vi "GetEdge DetectionResultValue.vi"(8 "error in (no error)":errorcluster, 9 "data":T2 {"Edge Information"."Distance (Real-World)" format="%.2f"; "Edge Information"."Location (Real-World)"."Y" format="%.2g"; "Edge Information"."Location (Real-World)"."X" format="%.2f"; "Edge Information"."Noise" format="%.2f"; "Edge Information"."Location (Pixel)"."Y" format="%.2g"; "Edge Information"."Location (Pixel)"."X" format="%.2f"; "Edge Information"."Strength" format="%.2f"; "Edge Information"."Distance (Pixel)" format="%.2f"}, 11 "Analysis_Edge Detection_Parameter":T3={"Edge Options"={"Edge Polarity"=0, "Kernel Size"=3, "Width"=5, "Minimum Edge Strength"=10.0, "Interpolation Type"=1, "Data Processing Method"=0}, "Process"=2, "Number of Matches Requested"=1, "ROI Descriptor"={"Global Rectangle"=[], "Contours"=[]}} {"Process" items=["Get First Edge", "Get First + Last Edge", "Get All Edges", "Get Best Edge"]; "Edge Options"."Data Processing Method" items=["Average", "Median"]; "Edge Options"."Interpolation Type" items=["Zero Order"=0, "Bilinear"=1, "Bilinear Fixed"=4]; "Edge Options"."Minimum Edge Strength" min=0.0 max=255.0 format="%.2g"; "Edge Options"."Width" min=1 step=2; "Edge Options"."Kernel Size" min=3 step=2; "Edge Options"."Edge Polarity" items=["All Edges", "Rising Edges", "Falling Edges"]}) -> (0 "error out":errorcluster, 3 "ResultValues":string[](array[string]))   [LabVIEW 2019]
uses:
  Controls/Edge Detection/Analysis_Edge Detection_Parameter.ctl
  <vilib>/vision/Measure.llb/Edge New.ctl
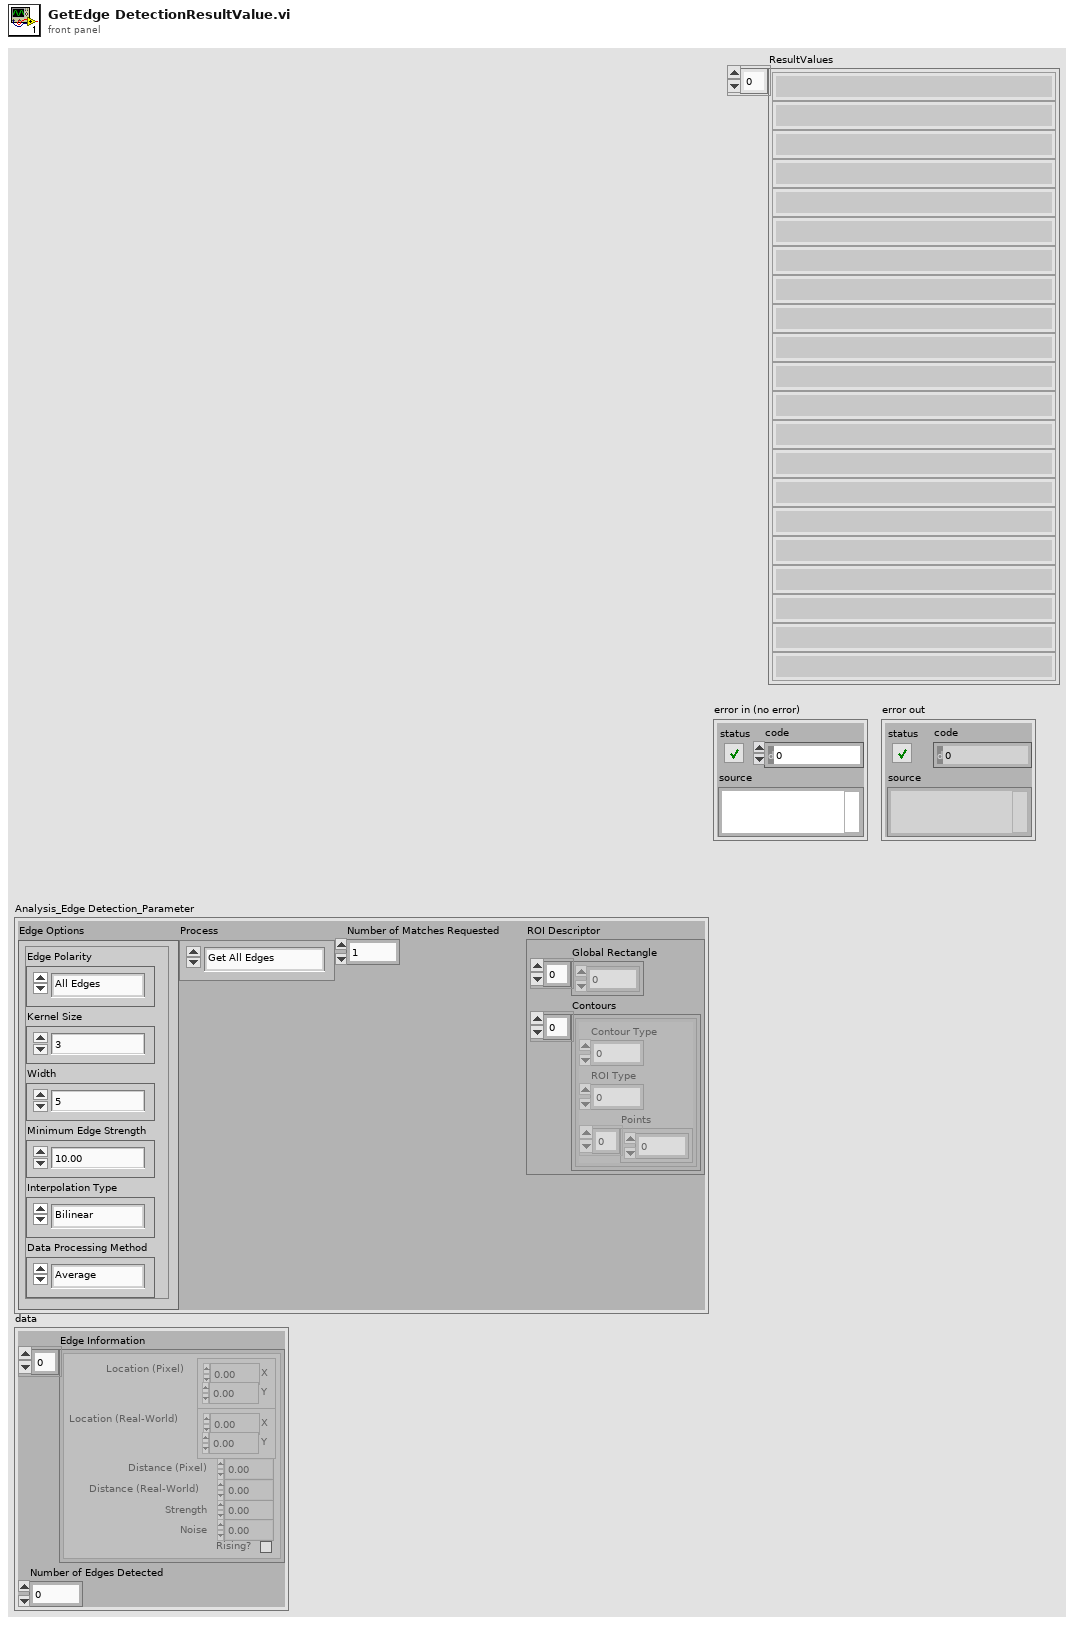
[diagram p1: front panel]
types:
  T1 = typedef "Edge New.ctl" = cluster{"Location (Pixel)":cluster{"X":sgl, "Y":sgl}, "Location (Real-World)":cluster{"X":sgl, "Y":sgl}, "Distance (Pixel)":dbl, "Distance (Real-World)":dbl, "Strength":dbl, "Noise":dbl, "Rising?":bool}
  T2 = cluster{"Edge Information":T1[], "Number of Edges Detected":i32}
  T3 = typedef "Analysis_Edge Detection_Parameter.ctl" = cluster{"Edge Options":cluster{"Edge Polarity":u16, "Kernel Size":u32, "Width":u32, "Minimum Edge Strength":dbl, "Interpolation Type":u16, "Data Processing Method":u16}, "Process":u16, "Number of Matches Requested":i32, "ROI Descriptor":cluster{"Global Rectangle":i32[], "Contours":cluster{"Contour Type":u32, "ROI Type":u32, "Points":i32[]}[]}}
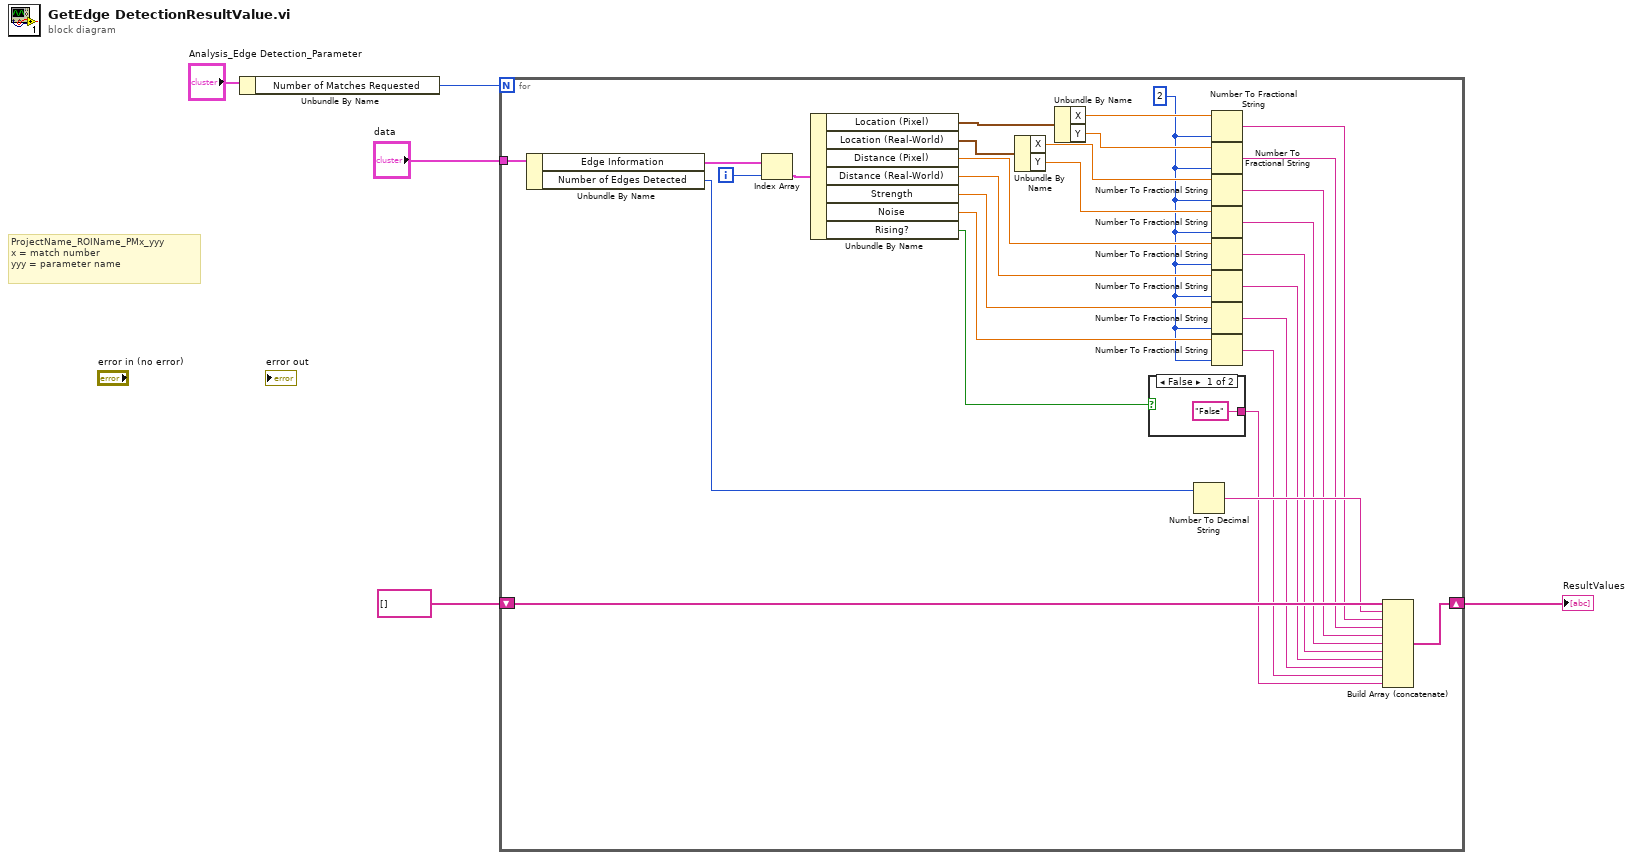
[diagram p0: block diagram]
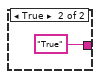
[diagram p2: hidden frame]
diagram:
  # "ProjectName_ROIName_PMx_yyy\nx = match number\nyyy = parameter name"
  n1 = Unbundle By Name("Analysis_Edge Detection_Parameter") -> ("Number of Matches Requested"=w2:i32)
  n2 = for {
    N: w2 -> [_]
    shift-right: [w8] -> w4
    shift-left: string[] [] -> [w18]
    tunnel: "data" -> [w34]
    i -> [w32]
    w6 = 2
    n3 = Unbundle By Name(w34) -> ("Edge Information"=w33:T1[], "Number of Edges Detected"=w30:i32)
    n4 = Index Array(array=w33, index=w32) -> (element=w31:T1)
    n5 = Unbundle By Name(w31) -> ("Location (Pixel)"=w29:cluster{"X":sgl, "Y":sgl}, "Location (Real-World)"=w28:cluster{"X":sgl, "Y":sgl}, "Distance (Pixel)"=w23:dbl, "Distance (Real-World)"=w22:dbl, "Strength"=w21:dbl, "Noise"=w20:dbl, "Rising?"=w19:bool)
    n6 = Unbundle By Name(w28) -> ("X"=w25:sgl, "Y"=w24:sgl)
    n7 = Unbundle By Name(w29) -> ("X"=w27:sgl, "Y"=w26:sgl)
    n8 = case shown="False" w19 {
      tunnel: ["False" "True"] -> w7
      frame False {
      }
      frame True {
      }
    }
    n9 = Number To Decimal String(number=w30) -> (decimal integer string=w17:string)  [unwired: 1 in]
    n10 = Number To Fractional String(number=w27, precision (6)=w6) -> (F-format string=w16:string)  [unwired: 2 in]
    n11 = Number To Fractional String(number=w26, precision (6)=w6) -> (F-format string=w15:string)  [unwired: 2 in]
    n12 = Number To Fractional String(number=w25, precision (6)=w6) -> (F-format string=w14:string)  [unwired: 2 in]
    n13 = Number To Fractional String(number=w24, precision (6)=w6) -> (F-format string=w13:string)  [unwired: 2 in]
    n14 = Number To Fractional String(number=w23, precision (6)=w6) -> (F-format string=w12:string)  [unwired: 2 in]
    n15 = Number To Fractional String(number=w22, precision (6)=w6) -> (F-format string=w11:string)  [unwired: 2 in]
    n16 = Number To Fractional String(number=w21, precision (6)=w6) -> (F-format string=w10:string)  [unwired: 2 in]
    n17 = Number To Fractional String(number=w20, precision (6)=w6) -> (F-format string=w9:string)  [unwired: 2 in]
    n18 = Build Array (concatenate)(w18, w17, w16, w15, w14, w13, w12, w11, w10, w9, w7) -> (w8:string[])
  }
  "ResultValues" <- w4
